vi "add_visa_in_error_in.vi"(0 "VI Ref In":refnum<vi>, 5 "Visa In Position":cluster{"Left":i32, "Top":i32}, 7 "Error In Position":cluster{"Left":i32, "Top":i32}, 11 "error in":errorcluster) -> (4 "VI Ref Out":refnum<vi>, 6 "VISA In Term":refnum<vi>, 8 "Error In Term":refnum<vi>, 15 "error out":errorcluster)   [LabVIEW 2018]
uses:
  Iternl/AddObj/AddControl/TypeDefinitions/bd_control_type.ctl
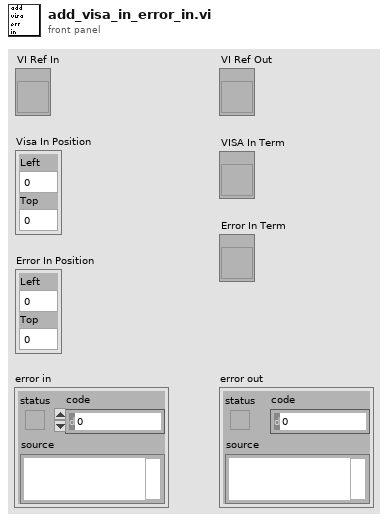
[diagram p1: front panel]
types:
  T1 = typedef "bd_control_type.ctl" = enum16{"Numeric", "Ring", "Boolean", "String", "VisaIn", "VisaOut", "Error In", "Error Out", "Array", "Waveform"}
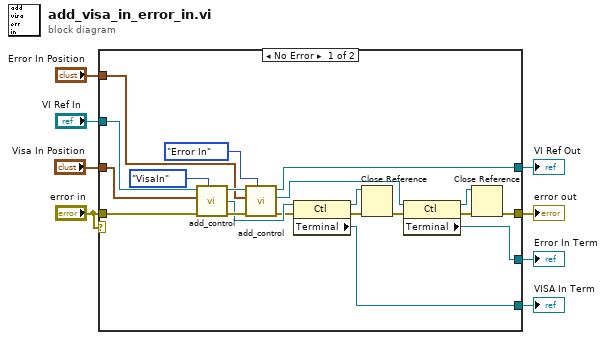
[diagram p0: block diagram]
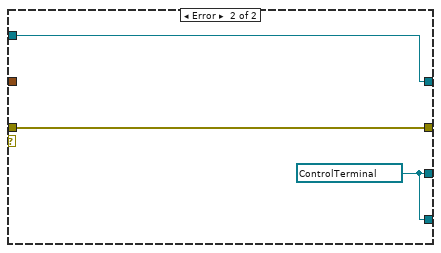
[diagram p2: hidden frame]
diagram:
  n1 = case shown="No Error" "error in" {
    tunnel: [w28 w31] -> w8
    tunnel: [w27 w30] -> w7
    tunnel: "VI Ref In" -> [w23 w30]
    tunnel: "Error In Position" -> [w22 _]
    tunnel: [w15 w29] -> w4
    tunnel: [w14 w29] -> w3
    tunnel: "Visa In Position" -> [w13 _]
    tunnel: "error in" -> [w12 w31]
    frame No Error {
      n2 = call "add_control.vi"("Add Control Type"=bd_control_type."VisaIn" ("Enum"), "error in (no error)"=w12, "BD Position"=w13, "VI Ref In"=w23) -> ("error out"=w24:errorcluster, "Control Ref Out"=w21:refnum<vi>, "VI Ref Out"=w26:refnum<vi>)  [unwired: 1 in, 4 out]
      n3 = call "add_control.vi"("Add Control Type"=bd_control_type."Error In" ("Enum"), "error in (no error)"=w24, "BD Position"=w22, "VI Ref In"=w26) -> ("error out"=w11:errorcluster, "Control Ref Out"=w20:refnum<vi>, "VI Ref Out"=w27:refnum<vi>)  [unwired: 1 in, 4 out]
      n4 = property class="Ctl"(reference=w21, error in=w11) -> (reference out=w17:refnum<vi>, error out=w16:errorcluster, "Terminal"=w15:refnum<vi>)
      n5 = Close Reference(reference=w17, error in (no error)=w16) -> (error out=w25:errorcluster)
      n6 = property class="Ctl"(reference=w20, error in=w25) -> (reference out=w19:refnum<vi>, error out=w18:errorcluster, "Terminal"=w14:refnum<vi>)
      n7 = Close Reference(reference=w19, error in (no error)=w18) -> (error out=w28:errorcluster)
    }
    frame Error {
      w29 = refnum<vi> refnum ("Terminal")
    }
  }
  "error out" <- w8
  "VI Ref Out" <- w7
  "VISA In Term" <- w4
  "Error In Term" <- w3
